vi "Load MICS Tables.vi"() -> ()   [LabVIEW 2010]
doc: "This function is an offline tool for importing MICS Command and Response Tables from Excel. \n\nInstructions\n1) Copy clipboard from Excel to Import Control.\n2) Run VI.\n3) Edit - Make Current Values Defaults.\n4) Save VI.\n5) Copy tables to new VIs."
panel:
  out "error out":errorcluster
  in  "error in":errorcluster
  in  "Table 2":string[][](table)=[["255", "0xFF", "COMMAND ACCEPTED", "The received command (identified in the response) was processed and performed without error. Any data to be returned as a result of the command completion is present in the response."], ["0", "0x00", "INVALID EXID", "The External ID contained in the command is for an external device the xPG has not been configured to process commands from."], ["1", "0x01", "INVALID COMMAND", "The Token in the received command is invalid/unknown to the xPG."], ["2", "0x02", "INVALID PARAM", "A parameter provided with the received command has been determined to be invalid and prohibits further processing of the command."], ["3", "0x03", "BUSY", "The xPG cannot execute the received command while in its present operational state.  Examples include: * Selecting program while stim on * Restoring program defaults while stim on * Writing to flash while stim on [CP commands] "], ["16", "0x10", "COMMAND NOT VALID WHILE IDLE", "The command is not valid when stimulation is not active.  (This code generally applies to commands that are used to modify stimulation.)"], ["17", "0x11", "COMMAND NOT VALID WHILE RAMPING", "The command is not valid when the xPG is ramping the stimulus amplitude immediately after turning stimulation on.  (This code generally applies to commands that are used to modify stimulation parameters)"], ["18", "0x12", "COMMAND LOCKED OUT (temporary)", "The command is temporarily locked out. (This code generally applies to commands that are used to modify stimulation, resulting in an increase in stimulation energy)"], ["19", "0x13", "DEPRECATED", ""], ["32", "0x20", "PROGRAM NOT VALID", "The command cannot be executed because the program definition is not valid.  A way to delete a program is to set it not valid.  Then when IPG returns valid programs bitmap it will not be listed as available."], ["33", "0x21", "PROGRAM DISABLED", "The command cannot be executed because the program definition has been disabled, due to a hardware issue."], ["34", "0x22", "BATTERY TOO LOW", "The xPG Stimulation command to turn stimulation on cannot be executed because the battery level is too low for safe stimulation.  IPG could have said battery was OK, but then dropped below threshold since having last sent status.  "], ["35", "0x23", "DEPRECATED –  Use 0x03 BUSY. ", ""], ["36", "0x24", "NO PROGRAM SELECTED", "The requested command (only in response to stim on) cannot be executed because no program is presently selected."], ["37", "0x25", "BOOST CONVERTER STARTUP FAILED", "Stimulation cannot be started because the high voltage boost converter did not initialize correctly."], ["38", "0x26", "PULSE GUARD CHECK FAILED", "Stimulation cannot be started because the pulse guard circuit check failed."], ["39", "0x27", "STIMULATION POWER ON FAILED", "Stimulation cannot be started because the stimulation chip failed to power up correctly."], ["40", "0x28", "ACTIVE RECOVERY DISABLED", "Stimulation cannot be started because automatic waveform adjustment failed."], ["41", "0x29", "DEPRECATED – Use 0x36 MOD VIOLATES ELECTRODE CHARGE DENSITY LIMIT", ""], ["42", "0x2A", "DEPRECATED – Use 0x02 INVALID PARAM.", ""], ["43", "0x2B", "DEPRECATED – USE 0x02 INVALID PARAM.", ""], ["44", "0x2C", "DEPRECATED – Use 0x02 INVALID PARAM.", ""], ["45", "0x2D", "DEPRECATED – Use 0x02 INVALID PARAM.", ""], ["46", "0x2E", "SETUP ERROR, BAD STIM ASIC READ-BACK", "While attempting to set-up the stim ASIC for output, the verification data read-back of certain registers did not match the set-up data. "], ["47", "0x2F", "SETUP ERROR, BAD POWER ASIC READ-BACK", "While attempting to configure the power ASIC, the verification data read-back of certain registers did not match the set-up data."], ["48", "0x30", "DEPRECATED – Not Used.", ""], ["49", "0x31", "ALL AMPLITUDES AT MINIMUM", "The Decrement Program Amplitude command cannot be executed because all pulse amplitudes are the minimum allowed setting."], ["50", "0x32", "ALL AMPLITUDES AT MAXIMUM", "The Increment Program Amplitude command cannot be executed because all pulse amplitudes are the maximum allowed setting."], ["51", "0x33", "PULSE NOT VALID", "The command to modify the specified pulse amplitude or pulse width cannot be executed because the pulse in not defined in the program that is running."], ["52", "0x34", "PULSE WIDTH EXCEEDS LIMITS", "The requested pulse width modification command cannot be executed because it would exceed the programmed pulse width limits for the specified pulse."], ["53", "0x35", "DEPRECATED - Use 0x02 INVALID PARAM.", ""], ["54", "0x36", "MOD VIOLATES ELECTRODE CHARGE DENSITY LIMIT", "The requested pulse output modification cannot be executed because it would violate the charge density limit for one or more of the selected electrode channels."], ["55", "0x37", "MOD VIOLATES ELECTRODE CURRENT DENSITY LIMIT", "The requested pulse output modification cannot be executed because it would violate the current density limit for one or more of the selected electrode channels."], ["56", "0x38", "PULSE WIDTH FREQUENCY CONFLICT", "* The requested pulse width increase cannot be executed because the program cannot be implemented at the specified program frequency. * The requested program frequency increase cannot be executed because the program cannot be implemented with the specified pulse widths. * The requested Test Pulse will not fit in the selected program period. * The requested pulse output requires active recovery, but the KrecsEnabledBitMap in the Pulse Constants is 0 (no krecs enabled). * The requested pulse output requires active recovery, but there are no krecs enabled (KrecsEnabledBitMap in Pulse Constants) that will fit the selected program period. "], ["57", "0x39", "DEPRECATED – Use PULSE WIDTH FREQUENCY CONFLICT", ""], ["58", "0x3A", "FREQUENCY MOD NOT ALLOWED", "The requested program frequency change is not allowed per the program definition.  (This could be because the specified frequency is not allowed or there is no frequency index lower or higher than the present index allowed.)"], ["59", "0x3B", "PULSE AMPLITUDE EXCEEDS LIMITS", "The requested pulse amplitude change cannot be executed because it would exceed the allowed limits for the specified pulse."], ["60", "0x3C", "DEPRECATED – Command n long exists", ""], ["64", "0x40", "TIMED OUT", "The operation requested timed out waiting for hardware to respond.  This response includes when an ADC read fails or when background impedance check fails to respond with a value."], ["85", "0x55", "CHARGING CONTROL ERROR", "An error occurred reading the temperature or battery level."], ["96", "0x60", "DATA CORRUPTED", "The requested Get Data command failed, or the requested data was detected as corrupt."], ["97", "0x61", "PROGRAM DEFINITION CORRUPTED", "The data integrity check for the program definition data for the requested program failed. IPG should set active error to PROGRAM DEFINITION CORRUPTED"], ["98", "0x62", "PROGRAM ACTIVE SETTINGS CORRUPTED", "The data integrity check for the active settings for the requested program failed.  IPG should set active error to PROGRAM ACTIVE SETTINGS CORRUPTED.  IPG will also return that active settings to default settings."], ["99", "0x63", "PROGRAM CONSTANTS CORRUPTED", "The data integrity check for the Program Constants data failed.  xPG should set active error to CRITICAL NV DATA CORRUPTED."], ["100", "0x64", "PULSE CONSTANTS CORRUPTED", "The data integrity check for the Pulse Constants data failed.  xPG should set active error to CRITICAL NV DATA CORRUPTED."], ["101", "0x65", "CHANNEL CALIBRATIONS CORRUPTED", "The data integrity check for the Channel Calibrations data failed.  xPG should set active error to CRITICAL NV DATA CORRUPTED."], ["102", "0x66", "LEAD LIMITS CORRUPTED", "The data integrity check for the Lead Limits data failed.  xPG should set active error to CRITICAL NV DATA CORRUPTED."], ["103", "0x67", "STIM ASIC HV CALIBRATIONS CORRUPTED", "The data integrity check for the Stim Asic HV Calibrations data failed.  xPG should set active error to CRITICAL NV DATA CORRUPTED."], ["104", "0x68", "RAMP TIME CORRUPTED", "The data integrity check for the Ramp Time failed.  xPG should set active error to CRITICAL NV DATA CORRUPTED."], ["105", "0x69", "DEPRECATED", ""], ["106", "0x6A", "DEPRECATED – Not Used", ""], ["112", "0x70", "FEATURE NOT ENABLED", "The requested feature is not presently enabled."], ["113", "0x71", "DEPRECATED - Use 0x02 INVALID PARAM.", ""], ["114", "0x72", "DEPRECATED - Use 0x02 INVALID PARAM.", ""], ["115", "0x73", "DEPRECATED – Use 0x03 BUSY.", ""], ["116", "0x74", "DEPRECATED – Use 0x38 PULSE WIDTH FREQUENCY CONFLICT", ""], ["117", "0x75", "DEPRECATED – Use 0x38 PULSE WIDTH FREQUENCY CONFLICT", ""], ["118", "0x76", "DEPRECATED – Use 0x38 PULSE WIDTH FREQUENCY CONFLICT", ""], ["119", "0x77", "WRITE FAILED", "The command failed while attempting to write data to memory or registers. Writes to flash shall use more specific error codes from the range below."], ["120", "0x78", "READ FAILED", "The command failed while attempting to read data to memory or registers. Reads to flash shall use more specific error codes from the range below."], ["121", "0x79", "DEPRECATED – Not Used", ""], ["128", "0x80", "DEPRECATED – Not Used", ""], ["129", "0x81", "BACKGROUND IMPEDANCE CHECK FAILED", "Pre-stimulation background impedance checks have failed.  This shall result in a Category 2 Error being reported."], ["130", "0x82", "BASIC OUTPUT CHECK FAILED", "Pre-stimulation basic output checks have failed.  This shall result in a Category 2 Error being reported."], ["131", "0x83", "STIM FAILED UNKNOWN SOFTWARE ERROR", "Stimulation has failed because of a software logic error.  Stimulation cannot be started."], ["132", "0x84", "STIMULATION FAILED – SEVERE ERROR EXISTS", "Stimulation has failed because a Category 1 error exists.  Stimulation cannot be started if such an error exists."], ["133", "0x85", "DEPRECATED – Not Used", ""], ["176", "0xB0", "FLASH ERROR INVALID ADDRESS", "Illegal flash address segment write.  The requested programming command failed while attempting to save data to the xPG’s non-volatile memory."], ["177", "0xB1", "FLASH ERROR SEGMENT BOUNDARY", "Requested flash address write overlaps segment boundary.  The requested programming command failed while attempting to save data to the xPG’s non-volatile memory."], ["178", "0xB2", "DEPRECATED – Use 0xB0 FLASH ERROR INVALID ADDRESS", "Invalid flash address reported while preparing for erasing segment.  The requested programming command failed while attempting to save data to the xPG’s non-volatile memory."], ["179", "0xB3", "FLASH ERASE ERROR FLASH CONTROLLER BUSY", "Flash controller unexpectedly reported busy while preparing for segment erase.  The requested programming command failed while attempting to save data to the xPG’s non-volatile memory."], ["180", "0xB4", "FLASH ERASE ERROR FLASH CONTROLLER SETUP", "Firmware setup error reported while preparing for segment erase.  The requested programming command failed while attempting to save data to the xPG’s non-volatile memory."], ["181", "0xB5", "FLASH ERASE ERROR TIMEOUT", "Busy bit timeout reported while waiting for segment erase. The requested programming command failed while attempting to save data to the xPG’s non-volatile memory."], ["182", "0xB6", "FLASH ERASE ERROR FAIL FLAG", "Fail flag set during segment erase.  The requested programming command failed while attempting to save data to the xPG’s non-volatile memory."], ["183", "0xB7", "FLASH ERASE ERROR ACCESS VIOLATION FLAG", "Access violation reported while attempting to erase flash.  The requested programming command failed while attempting to save data to the xPG’s non-volatile memory."], ["184", "0xB8", "FLASH ERASE ERROR BAD ERASE", "Segment not erased and segment erase reported as completed.  The requested programming command failed while attempting to save data to the xPG’s non-volatile memory."], ["192", "0xC0", "DEPRECATED – Use 0xB0 FLASH ERROR INVALID ADDRESS", ""], ["193", "0xC1", "FLASH WRITE ERROR FLASH CONTROLLER BUSY", "The flash controller reports unexpectedly busy while preparing for block write.  The requested programming command failed while attempting to save data to the xPG’s non-volatile memory."], ["194", "0xC2", "FLASH WRITE ERROR FLASH CONTROLLER SETUP", "A firmware setup error occurred while preparing for block write.  The requested programming command failed while attempting to save data to the xPG’s non-volatile memory."], ["195", "0xC3", "FLASH WORD WRITE ERROR TIMEOUT", "Wait bit timeout occurred while writing word to flash memory.  The requested programming command failed while attempting to save data to the xPG’s non-volatile memory."], ["196", "0xC4", "FLASH  WORD WRITE ERROR FAIL FLAG", "Flash fail flag set while writing word to flash memory.  The requested programming command failed while attempting to save data to the xPG’s non-volatile memory."], ["197", "0xC5", "FLASH WORD WRITE ERROR ACCESS VIOLATION", "Access violation reported while writing word to flash memory.  The requested programming command failed while attempting to save data to the xPG’s non-volatile memory."], ["198", "0xC6", "FLASH BLOCK WRITE ERROR TIMEOUT", "Wait bit timeout occurred while writing block to flash memory.  The requested programming command failed while attempting to save data to the xPG’s non-volatile memory."], ["199", "0xC7", "FLASH  BLOCK WRITE ERROR FAIL FLAG", "Flash fail flag set while writing block to flash memory.  The requested programming command failed while attempting to save data to the xPG’s non-volatile memory."], ["200", "0xC8", "FLASH BLOCK WRITE ERROR ACCESS VIOLATION", "Access violation reported while writing block to flash memory.  The requested programming command failed while attempting to save data to the xPG’s non-volatile memory."], ["201", "0xC9", "FLASH WRITE ERROR BAD WRITE", "After segment write completed, the flash destination data did not match the source data.  The requested programming command failed while attempting to save data to the xPG’s non-volatile memory."], ["202", "0xCA", "RESERVED – Not Used.", ""], ["203", "0xCB", "RESERVED – Not Used.", ""], ["204", "0xCC", "RESERVED – Not Used.", ""], ["205", "0xCD", "RESERVED – Not Used.", ""], ["206", "0xCE", "RESERVED – Not Used.", ""], ["207", "0xCF", "RESERVED – Not Used.", ""], ["-1", "Default", "ANY ERROR NOT LISTED HEREIN", "Undefined and unexpected.   "]]
  in  "Excel Clipboard to Import 2":string="255\t0xFF\tCOMMAND ACCEPTED\tThe received command (identified in the response) was processed and performed without error. Any data to be returned as a result of the command completion is present in the response.\n0\t0x00\tINVALID EXID\tThe External ID contained in the command is for an external device the xPG has not been configured to process commands from.\n1\t0x01\tINVALID COMMAND\tThe Token in the received command is invalid/unknown to the xPG.\n2\t0x02\tINVALID PARAM\tA parameter provided with the received command has been determined to be invalid and prohibits further processing of the command.\n3\t0x03\tBUSY\tThe xPG cannot execute the received command while in its present operational state.  Examples include: * Selecting program while stim on * Restoring program defaults while stim on * Writing to flash while stim on [CP commands] \n16\t0x10\tCOMMAND NOT VALID WHILE IDLE\tThe command is not valid when stimulation is not active.  (This code generally applies to commands that are used to modify stimulation.)\n17\t0x11\tCOMMAND NOT VALID WHILE RAMPING\tThe command is not valid when the xPG is ramping the stimulus amplitude immediately after turning stimulation on.  (This code generally applies to commands that are used to modify stimulation parameters)\n18\t0x12\tCOMMAND LOCKED OUT (temporary)\tThe command is temporarily locked out. (This code generally applies to commands that are used to modify stimulation, resulting in an increase in stimulation energy)\n19\t0x13\tDEPRECATED\t\n32\t0x20\tPROGRAM NOT VALID\tThe command cannot be executed because the program definition is not valid.  A way to delete a program is to set it not valid.  Then when IPG returns valid programs bitmap it will not be listed as available.\n33\t0x21\tPROGRAM DISABLED\tThe command cannot be executed because the program definition has been disabled, due to a hardware issue.\n34\t0x22\tBATTERY TOO LOW\tThe xPG Stimulation command to turn stimulation on cannot be executed because the battery level is too low for safe stimulation.  IPG could have said battery was OK, but then dropped below threshold since having last sent status.  \n35\t0x23\tDEPRECATED –  Use 0x03 BUSY. \t\n36\t0x24\tNO PROGRAM SELECTED\tThe requested command (only in response to stim on) cannot be executed because no program is presently selected.\n37\t0x25\tBOOST CONVERTER STARTUP FAILED\tStimulation cannot be started because the high voltage boost converter did not initialize correctly.\n38\t0x26\tPULSE GUARD CHECK FAILED\tStimulation cannot be started because the pulse guard circuit check failed.\n39\t0x27\tSTIMULATION POWER ON FAILED\tStimulation cannot be started because the stimulation chip failed to power up correctly.\n40\t0x28\tACTIVE RECOVERY DISABLED\tStimulation cannot be started because automatic waveform adjustment failed.\n41\t0x29\tDEPRECATED – Use 0x36 MOD VIOLATES ELECTRODE CHARGE DENSITY LIMIT\t\n42\t0x2A\tDEPRECATED – Use 0x02 INVALID PARAM.\t\n43\t0x2B\tDEPRECATED – USE 0x02 INVALID PARAM.\t\n44\t0x2C\tDEPRECATED – Use 0x02 INVALID PARAM.\t\n45\t0x2D\tDEPRECATED – Use 0x02 INVALID PARAM.\t\n46\t0x2E\tSETUP ERROR, BAD STIM ASIC READ-BACK\tWhile attempting to set-up the stim ASIC for output, the verification data read-back of certain registers did not match the set-up data. \n47\t0x2F\tSETUP ERROR, BAD POWER ASIC READ-BACK\tWhile attempting to configure the power ASIC, the verification data read-back of certain registers did not match the set-up data.\n48\t0x30\tDEPRECATED – Not Used.\t\n49\t0x31\tALL AMPLITUDES AT MINIMUM\tThe Decrement Program Amplitude command cannot be executed because all pulse amplitudes are the minimum allowed setting.\n50\t0x32\tALL AMPLITUDES AT MAXIMUM\tThe Increment Program Amplitude command cannot be executed because all pulse amplitudes are the maximum allowed setting.\n51\t0x33\tPULSE NOT VALID\tThe command to modify the specified pulse amplitude or pulse width cannot be executed because the pulse in not defined in the program that is running.\n52\t0x34\tPULSE WIDTH EXCEEDS LIMITS\tThe requested pulse width modification command cannot be executed because it would exceed the programmed pulse width limits for the specified pulse.\n53\t0x35\tDEPRECATED - Use 0x02 INVALID PARAM.\t\n54\t0x36\tMOD VIOLATES ELECTRODE CHARGE DENSITY LIMIT\tThe requested pulse output modification cannot be executed because it would violate the charge density limit for one or more of the selected electrode channels.\n55\t0x37\tMOD VIOLATES ELECTRODE CURRENT DENSITY LIMIT\tThe requested pulse output modification cannot be executed because it would violate the current density limit for one or more of the selected electrode channels.\n56\t0x38\tPULSE WIDTH FREQUENCY CONFLICT\t* The requested pulse width increase cannot be executed because the program cannot be implemented at the specified program frequency. * The requested program frequency increase cannot be executed because the program cannot be implemented with the specified pulse widths. * The requested Test Pulse will not fit in the selected program period. * The requested pulse output requires active recovery, but the KrecsEnabledBitMap in the Pulse Constants is 0 (no krecs enabled). * The requested pulse output requires active recovery, but there are no krecs enabled (KrecsEnabledBitMap in Pulse Constants) that will fit the selected program period. \n57\t0x39\tDEPRECATED – Use PULSE WIDTH FREQUENCY CONFLICT\t\n58\t0x3A\tFREQUENCY MOD NOT ALLOWED\tThe requested program frequency change is not allowed per the program definition.  (This could be because the specified frequency is not allowed or there is no frequency index lower or higher than the present index allowed.)\n59\t0x3B\tPULSE AMPLITUDE EXCEEDS LIMITS\tThe requested pulse amplitude change cannot be executed because it would exceed the allowed limits for the specified pulse.\n60\t0x3C\tDEPRECATED – Command n long exists\t\n64\t0x40\tTIMED OUT\tThe operation requested timed out waiting for hardware to respond.  This response includes when an ADC read fails or when background impedance check fails to respond with a value.\n85\t0x55\tCHARGING CONTROL ERROR\tAn error occurred reading the temperature or battery level.\n96\t0x60\tDATA CORRUPTED\tThe requested Get Data command failed, or the requested data was detected as corrupt.\n97\t0x61\tPROGRAM DEFINITION CORRUPTED\tThe data integrity check for the program definition data for the requested program failed. IPG should set active error to PROGRAM DEFINITION CORRUPTED\n98\t0x62\tPROGRAM ACTIVE SETTINGS CORRUPTED\tThe data integrity check for the active settings for the requested program failed.  IPG should set active error to PROGRAM ACTIVE SETTINGS CORRUPTED.  IPG will also return that active settings to default settings.\n99\t0x63\tPROGRAM CONSTANTS CORRUPTED\tThe data integrity check for the Program Constants data failed.  xPG should set active error to CRITICAL NV DATA CORRUPTED.\n100\t0x64\tPULSE CONSTANTS CORRUPTED\tThe data integrity check for the Pulse Constants data failed.  xPG should set active error to CRITICAL NV DATA CORRUPTED.\n101\t0x65\tCHANNEL CALIBRATIONS CORRUPTED\tThe data integrity check for the Channel Calibrations data failed.  xPG should set active error to CRITICAL NV DATA CORRUPTED.\n102\t0x66\tLEAD LIMITS CORRUPTED\tThe data integrity check for the Lead Limits data failed.  xPG should set active error to CRITICAL NV DATA CORRUPTED.\n103\t0x67\tSTIM ASIC HV CALIBRATIONS CORRUPTED\tThe data integrity check for the Stim Asic HV Calibrations data failed.  xPG should set active error to CRITICAL NV DATA CORRUPTED.\n104\t0x68\tRAMP TIME CORRUPTED\tThe data integrity check for the Ramp Time failed.  xPG should set active error to CRITICAL NV DATA CORRUPTED.\n105\t0x69\tDEPRECATED\t\n106\t0x6A\tDEPRECATED – Not Used\t\n112\t0x70\tFEATURE NOT ENABLED\tThe requested feature is not presently enabled.\n113\t0x71\tDEPRECATED - Use 0x02 INVALID PARAM.\t\n114\t0x72\tDEPRECATED - Use 0x02 INVALID PARAM.\t\n115\t0x73\tDEPRECATED – Use 0x03 BUSY.\t\n116\t0x74\tDEPRECATED – Use 0x38 PULSE WIDTH FREQUENCY CONFLICT\t\n117\t0x75\tDEPRECATED – Use 0x38 PULSE WIDTH FREQUENCY CONFLICT\t\n118\t0x76\tDEPRECATED – Use 0x38 PULSE WIDTH FREQUENCY CONFLICT\t\n119\t0x77\tWRITE FAILED\tThe command failed while attempting to write data to memory or registers. Writes to flash shall use more specific error codes from the range below.\n120\t0x78\tREAD FAILED\tThe command failed while attempting to read data to memory or registers. Reads to flash shall use more specific error codes from the range below.\n121\t0x79\tDEPRECATED – Not Used\t\n128\t0x80\tDEPRECATED – Not Used\t\n129\t0x81\tBACKGROUND IMPEDANCE CHECK FAILED\tPre-stimulation background impedance checks have failed.  This shall result in a Category 2 Error being reported.\n130\t0x82\tBASIC OUTPUT CHECK FAILED\tPre-stimulation basic output checks have failed.  This shall result in a Category 2 Error being reported.\n131\t0x83\tSTIM FAILED UNKNOWN SOFTWARE ERROR\tStimulation has failed because of a software logic error.  Stimulation cannot be started.\n132\t0x84\tSTIMULATION FAILED – SEVERE ERROR EXISTS\tStimulation has failed because a Category 1 error exists.  Stimulation cannot be started if such an error exists.\n133\t0x85\tDEPRECATED – Not Used\t\n176\t0xB0\tFLASH ERROR INVALID ADDRESS\tIllegal flash address segment write.  The requested programming command failed while attempting to save data to the xPG’s non-volatile memory.\n177\t0xB1\tFLASH ERROR SEGMENT BOUNDARY\tRequested flash address write overlaps segment boundary.  The requested programming command failed while attempting to save data to the xPG’s non-volatile memory.\n178\t0xB2\tDEPRECATED – Use 0xB0 FLASH ERROR INVALID ADDRESS\tInvalid flash address reported while preparing for erasing segment.  The requested programming command failed while attempting to save data to the xPG’s non-volatile memory.\n179\t0xB3\tFLASH ERASE ERROR FLASH CONTROLLER BUSY\tFlash controller unexpectedly reported busy while preparing for segment erase.  The requested programming command failed while attempting to save data to the xPG’s non-volatile memory.\n180\t0xB4\tFLASH ERASE ERROR FLASH CONTROLLER SETUP\tFirmware setup error reported while preparing for segment erase.  The requested programming command failed while attempting to save data to the xPG’s non-volatile memory.\n181\t0xB5\tFLASH ERASE ERROR TIMEOUT\tBusy bit timeout reported while waiting for segment erase. The requested programming command failed while attempting to save data to the xPG’s non-volatile memory.\n182\t0xB6\tFLASH ERASE ERROR FAIL FLAG\tFail flag set during segment erase.  The requested programming command failed while attempting to save data to the xPG’s non-volatile memory.\n183\t0xB7\tFLASH ERASE ERROR ACCESS VIOLATION FLAG\tAccess violation reported while attempting to erase flash.  The requested programming command failed while attempting to save data to the xPG’s non-volatile memory.\n184\t0xB8\tFLASH ERASE ERROR BAD ERASE\tSegment not erased and segment erase reported as completed.  The requested programming command failed while attempting to save data to the xPG’s non-volatile memory.\n192\t0xC0\tDEPRECATED – Use 0xB0 FLASH ERROR INVALID ADDRESS\t\n193\t0xC1\tFLASH WRITE ERROR FLASH CONTROLLER BUSY\tThe flash controller reports unexpectedly busy while preparing for block write.  The requested programming command failed while attempting to save data to the xPG’s non-volatile memory.\n194\t0xC2\tFLASH WRITE ERROR FLASH CONTROLLER SETUP\tA firmware setup error occurred while preparing for block write.  The requested programming command failed while attempting to save data to the xPG’s non-volatile memory.\n195\t0xC3\tFLASH WORD WRITE ERROR TIMEOUT\tWait bit timeout occurred while writing word to flash memory.  The requested programming command failed while attempting to save data to the xPG’s non-volatile memory.\n196\t0xC4\tFLASH  WORD WRITE ERROR FAIL FLAG\tFlash fail flag set while writing word to flash memory.  The requested programming command failed while attempting to save data to the xPG’s non-volatile memory.\n197\t0xC5\tFLASH WORD WRITE ERROR ACCESS VIOLATION\tAccess violation reported while writing word to flash memory.  The requested programming command failed while attempting to save data to the xPG’s non-volatile memory.\n198\t0xC6\tFLASH BLOCK WRITE ERROR TIMEOUT\tWait bit timeout occurred while writing block to flash memory.  The requested programming command failed while attempting to save data to the xPG’s non-volatile memory.\n199\t0xC7\tFLASH  BLOCK WRITE ERROR FAIL FLAG\tFlash fail flag set while writing block to flash memory.  The requested programming command failed while attempting to save data to the xPG’s non-volatile memory.\n200\t0xC8\tFLASH BLOCK WRITE ERROR ACCESS VIOLATION\tAccess violation reported while writing block to flash memory.  The requested programming command failed while attempting to save data to the xPG’s non-volatile memory.\n201\t0xC9\tFLASH WRITE ERROR BAD WRITE\tAfter segment write completed, the flash destination data did not match the source data.  The requested programming command failed while attempting to save data to the xPG’s non-volatile memory.\n202\t0xCA\tRESERVED – Not Used.\t\n203\t0xCB\tRESERVED – Not Used.\t\n204\t0xCC\tRESERVED – Not Used.\t\n205\t0xCD\tRESERVED – Not Used.\t\n206\t0xCE\tRESERVED – Not Used.\t\n207\t0xCF\tRESERVED – Not Used.\t\n-1\tDefault\tANY ERROR NOT LISTED HEREIN\tUndefined and unexpected.   \n"
  in  "Excel Clipboard1 to Import 1":string="1\t0x0001\tGet xPG Status\tTKN_GET_XPG_STATUS\n2\t0x0002\txPG Stimulation\tTKN_XPG_STIMULATION\n3\t0x0003\tSelect Program\tTKN_SELECT_PROGRAM\n4\t0x0004\tIncrement Program Amplitude\tTKN_INC_PRGM_AMPL\n5\t0x0005\tDecrement Program Amplitude\tTKN_DEC_PRGM_AMPL\n6\t0x0006\tGet PoP Constants\tTKN_GET_POP_CONST\n7\t0x0007\tGet PPC Constants\tTKN_GET_PPC CONST\n8\t0x0008\tGet Program Names\tTKN_GET_PRGM_NAMES\n9\t0x0009\tSet Pulse Amplitude\tTKN_SET_PULSE_AMPL\n10\t0x000A\tIncrement Pulse Amplitude\tTKN_INC_PULSE_AMPL\n11\t0x000B\tDecrement Pulse Amplitude\tTKN_DEC_PULSE_AMPL\n12\t0x000C\tGet Pulse Widths\tTKN_GET_PULSE_WIDTHS\n13\t0x000D\tSet Pulse Widths\tTKN_SET_PULSE_WIDTH\n14\t0x000E\tIncrement Pulse Width\tTKN_INC_PULSE_WIDTH\n15\t0x000F\tDecrement Pulse Width\tTKN_DEC_PULSE_WIDTH\n16\t0x0010\tGet Program Frequency\tTKN_GET_PRGM_FREQ\n17\t0x0011\tSet Program Frequency\tTKN_SET_PRGM_FREQ\n18\t0x0012\tIncrement Program Frequency\tTKN_INC_PRGM_FREQ\n19\t0x0013\tDecrement Program Frequency\tTKN_DEC_PRGM_FREQ\n20\t0x0014\tInject Event\tTKN_INJECT_EVENT\n21\t0x0015\tCharging Control\tTKN_CHARGING_CONTROL\n22\t0x0016\tGet xPG Identity\tTKN_GET_XPG_IDENTITY\n23\t0x0017\tSet xPG Identity\tTKN_SET_XPG_IDENTITY\n24\t0x0018\tRestore Program Defaults\tTKN_RESTORE_DEFAULTS\n25\t0x0019\tGet Program Definition\tTKN_GET_PRGM_DEF\n26\t0x001A\tSet Program Definition\tTKN_SET_PRGM_DEF\n27\t0x001B\tGet Program Constants\tTKN_GET_PRGM_CONST\n28\t0x001C\tSet Program Constants\tTKN_SET_PRGM_CONST\n29\t0x001D\tGet Configurable Device Parameters\tTKN_GET_CONFIG_PARAMS\n30\t0x001E\tSet Configurable Device Parameters\tTKN_SET_CONFIG_PARAMS\n31\t0x001F\tGet Pulse Constants\tTKN_GET_PULSE_CONSTANTS\n32\t0x0020\tSet Pulse Constants\tTKN_SET_PULSE_CONSTANTS\n33\t0x0021\tGet Lead Limits\tTKN_GET_LEAD_LIMITS\n34\t0x0022\tSet Lead Limits\tTKN_SET_LEAD_LIMITS\n35\t0x0023\tGet Channel Calibrations\tTKN_GET_CHANNEL_CALS\n36\t0x0024\tSet Channel Calibrations\tTKN_SET_CHANNEL_CALS\n37\t0x0025\t(reserved)\tRESERVED_37\n38\t0x0026\t(reserved)\tRESERVED_38\n39\t0x0027\t(reserved)\tRESERVED_39\n40\t0x0028\t(reserved)\tRESERVED_40\n41\t0x0029\t(reserved)\tRESERVED_41\n42\t0x002A\t(reserved)\tRESERVED_42\n43\t0x002B\tGet Stim Asic HV Calibrations\tTKN_GET_HV_CALS\n44\t0x002C\tSet Stim Asic HV Calibrations\tTKN_SET_HV_CALS\n45\t0x002D\t(reserved)\tRESERVED_45\n46\t0x002E\t(reserved)\tRESERVED_46\n47\t0x002F\tGet CP Data\tTKN_GET_CP_DATA\n48\t0x0030\tSet CP Data\tTKN_SET_CP_DATA\n49\t0x0031\tClear Log\tTKN_CLEAR_LOG\n50\t0x0032\tRead Log\tTKN_READ_LOG\n51\t0x0033\tAppend Log\tTKN_APPEND_LOG\n52\t0x0034\t(reserved)\tRESERVED_52\n53\t0x0035\t(reserved)\tRESERVED_53\n54\t0x0036\tImpedance Measurement\tTKN_IMP_MEAS\n55\t0x0037\tEnter Storage Mode\tTKN_STORAGE\n56\t0x0038\tEcho Short\tTKN_ECHO_SHORT\n57\t0x0039\tEcho Long\tTKN_ECHO_LONG\n58\t0x003A\tGet General Calibration\tTKN_GET_GEN_CAL\n59\t0x003B\tSet General Calibration\tTKN_SET_GEN_CAL\n60\t0x003C\tGet Trim List\tTKN_GET_TRIM_LIST\n61\t0x003D\tSet Trim List\tTKN_SET_TRIM_LIST\n62\t0x003E\tGet Counter\tTKN_GET_COUNTER\n63\t0x003F\tSet Counter\tTKN_SET_COUNTER\n64\t0x0040\tGet Test Stimulation\tTKN_GET_TEST_STIM\n65\t0x0041\tSet Test Stimulation\tTKN_SET_TEST_STIM\n66\t0x0042\tGet Titration Stimulation\tTKN_GET_TITR_STIM\n67\t0x0043\tSet Titration Stimulation\tTKN_SET_TITR_STIM\n68\t0x0044\tGet Ramp Time\tTKN_GET_RAMP_TIME\n69\t0x0045\tSet Ramp Time\tTKN_SET_RAMP_TIME\n70\t0x0046\tGet VBAT\tTKN_GET_VBAT\n71\t0x0047\tSet Software Description Block\tTKN_SET_SDB\n72\t0x0048\tGet Software Description Block\tTKN_GET_SDB\n73\t0x0049\tWrite Memory\tTKN_WRITE_MEMORY\n74\t0x004A\tRead Memory\tTKN_READ_MEMORY\n75\t0x004B\tReset xPG\tTKN_RESET\n76\t0x004C\tErase Flash Block\tTKN_ERASE_FLASH_BLOCK\n77\t0x004D\tWrite Vectors\tTKN_WRITE_VECTORS\n78\t0x004E\tRead Vectors\tTKN_READ_VECTORS\n79\t0x004F\tDiagnostic Data\tTKN_DIAG_DATA\n80\t0x0050\tSet Background Impedance\tTKN_SET_BG_IMPEDANCE\n81\t0x0051\tGet Background Impedance\tTKN_GET_BG_IMPEDANCE\n82\t0x0052\tSet Test Waveform\tTKN_SET_TEST_WAVEFORM\n83\t0x0053\tCalibrate Channel\tTKN_CALIBRATE_CHANNEL\n84\t0x0054\tGet Log Range\tTKN_GET_LOG_RANGE\n85\t0x0055\t(reserved)\tRESERVED_85\n86\t0x0056\t(reserved)\tRESERVED_86\n87\t0x0057\tMICS Options\tTKN_MICS_OPTIONS\n88\t0x0058\tPair PPC\tTKN_PAIR_PPC\n89\t0x0059\tPair PoP\tTKN_PAIR_POP\n90\t0x005A\tStop Bootloader\tTKN_STOP_BOOTLOADER\n91\t0x005B\tTune MICS\tTKN_MICS_TUNE\n92\t0x005C\tMICS Diagnostics\tTKN_MICS_DIAGNOSTICS\n32682\t0x7FAA\tUndefined\tTKN_UNDEFINED\n"
  in  "Table 1":string[][](table)=[["1", "0x0001", "Get xPG Status", "TKN_GET_XPG_STATUS"], ["2", "0x0002", "xPG Stimulation", "TKN_XPG_STIMULATION"], ["3", "0x0003", "Select Program", "TKN_SELECT_PROGRAM"], ["4", "0x0004", "Increment Program Amplitude", "TKN_INC_PRGM_AMPL"], ["5", "0x0005", "Decrement Program Amplitude", "TKN_DEC_PRGM_AMPL"], ["6", "0x0006", "Get PoP Constants", "TKN_GET_POP_CONST"], ["7", "0x0007", "Get PPC Constants", "TKN_GET_PPC CONST"], ["8", "0x0008", "Get Program Names", "TKN_GET_PRGM_NAMES"], ["9", "0x0009", "Set Pulse Amplitude", "TKN_SET_PULSE_AMPL"], ["10", "0x000A", "Increment Pulse Amplitude", "TKN_INC_PULSE_AMPL"], ["11", "0x000B", "Decrement Pulse Amplitude", "TKN_DEC_PULSE_AMPL"], ["12", "0x000C", "Get Pulse Widths", "TKN_GET_PULSE_WIDTHS"], ["13", "0x000D", "Set Pulse Widths", "TKN_SET_PULSE_WIDTH"], ["14", "0x000E", "Increment Pulse Width", "TKN_INC_PULSE_WIDTH"], ["15", "0x000F", "Decrement Pulse Width", "TKN_DEC_PULSE_WIDTH"], ["16", "0x0010", "Get Program Frequency", "TKN_GET_PRGM_FREQ"], ["17", "0x0011", "Set Program Frequency", "TKN_SET_PRGM_FREQ"], ["18", "0x0012", "Increment Program Frequency", "TKN_INC_PRGM_FREQ"], ["19", "0x0013", "Decrement Program Frequency", "TKN_DEC_PRGM_FREQ"], ["20", "0x0014", "Inject Event", "TKN_INJECT_EVENT"], ["21", "0x0015", "Charging Control", "TKN_CHARGING_CONTROL"], ["22", "0x0016", "Get xPG Identity", "TKN_GET_XPG_IDENTITY"], ["23", "0x0017", "Set xPG Identity", "TKN_SET_XPG_IDENTITY"], ["24", "0x0018", "Restore Program Defaults", "TKN_RESTORE_DEFAULTS"], ["25", "0x0019", "Get Program Definition", "TKN_GET_PRGM_DEF"], ["26", "0x001A", "Set Program Definition", "TKN_SET_PRGM_DEF"], ["27", "0x001B", "Get Program Constants", "TKN_GET_PRGM_CONST"], ["28", "0x001C", "Set Program Constants", "TKN_SET_PRGM_CONST"], ["29", "0x001D", "Get Configurable Device Parameters", "TKN_GET_CONFIG_PARAMS"], ["30", "0x001E", "Set Configurable Device Parameters", "TKN_SET_CONFIG_PARAMS"], ["31", "0x001F", "Get Pulse Constants", "TKN_GET_PULSE_CONSTANTS"], ["32", "0x0020", "Set Pulse Constants", "TKN_SET_PULSE_CONSTANTS"], ["33", "0x0021", "Get Lead Limits", "TKN_GET_LEAD_LIMITS"], ["34", "0x0022", "Set Lead Limits", "TKN_SET_LEAD_LIMITS"], ["35", "0x0023", "Get Channel Calibrations", "TKN_GET_CHANNEL_CALS"], ["36", "0x0024", "Set Channel Calibrations", "TKN_SET_CHANNEL_CALS"], ["37", "0x0025", "(reserved)", "RESERVED_37"], ["38", "0x0026", "(reserved)", "RESERVED_38"], ["39", "0x0027", "(reserved)", "RESERVED_39"], ["40", "0x0028", "(reserved)", "RESERVED_40"], ["41", "0x0029", "(reserved)", "RESERVED_41"], ["42", "0x002A", "(reserved)", "RESERVED_42"], ["43", "0x002B", "Get Stim Asic HV Calibrations", "TKN_GET_HV_CALS"], ["44", "0x002C", "Set Stim Asic HV Calibrations", "TKN_SET_HV_CALS"], ["45", "0x002D", "(reserved)", "RESERVED_45"], ["46", "0x002E", "(reserved)", "RESERVED_46"], ["47", "0x002F", "Get CP Data", "TKN_GET_CP_DATA"], ["48", "0x0030", "Set CP Data", "TKN_SET_CP_DATA"], ["49", "0x0031", "Clear Log", "TKN_CLEAR_LOG"], ["50", "0x0032", "Read Log", "TKN_READ_LOG"], ["51", "0x0033", "Append Log", "TKN_APPEND_LOG"], ["52", "0x0034", "(reserved)", "RESERVED_52"], ["53", "0x0035", "(reserved)", "RESERVED_53"], ["54", "0x0036", "Impedance Measurement", "TKN_IMP_MEAS"], ["55", "0x0037", "Enter Storage Mode", "TKN_STORAGE"], ["56", "0x0038", "Echo Short", "TKN_ECHO_SHORT"], ["57", "0x0039", "Echo Long", "TKN_ECHO_LONG"], ["58", "0x003A", "Get General Calibration", "TKN_GET_GEN_CAL"], ["59", "0x003B", "Set General Calibration", "TKN_SET_GEN_CAL"], ["60", "0x003C", "Get Trim List", "TKN_GET_TRIM_LIST"], ["61", "0x003D", "Set Trim List", "TKN_SET_TRIM_LIST"], ["62", "0x003E", "Get Counter", "TKN_GET_COUNTER"], ["63", "0x003F", "Set Counter", "TKN_SET_COUNTER"], ["64", "0x0040", "Get Test Stimulation", "TKN_GET_TEST_STIM"], ["65", "0x0041", "Set Test Stimulation", "TKN_SET_TEST_STIM"], ["66", "0x0042", "Get Titration Stimulation", "TKN_GET_TITR_STIM"], ["67", "0x0043", "Set Titration Stimulation", "TKN_SET_TITR_STIM"], ["68", "0x0044", "Get Ramp Time", "TKN_GET_RAMP_TIME"], ["69", "0x0045", "Set Ramp Time", "TKN_SET_RAMP_TIME"], ["70", "0x0046", "Get VBAT", "TKN_GET_VBAT"], ["71", "0x0047", "Set Software Description Block", "TKN_SET_SDB"], ["72", "0x0048", "Get Software Description Block", "TKN_GET_SDB"], ["73", "0x0049", "Write Memory", "TKN_WRITE_MEMORY"], ["74", "0x004A", "Read Memory", "TKN_READ_MEMORY"], ["75", "0x004B", "Reset xPG", "TKN_RESET"], ["76", "0x004C", "Erase Flash Block", "TKN_ERASE_FLASH_BLOCK"], ["77", "0x004D", "Write Vectors", "TKN_WRITE_VECTORS"], ["78", "0x004E", "Read Vectors", "TKN_READ_VECTORS"], ["79", "0x004F", "Diagnostic Data", "TKN_DIAG_DATA"], ["80", "0x0050", "Set Background Impedance", "TKN_SET_BG_IMPEDANCE"], ["81", "0x0051", "Get Background Impedance", "TKN_GET_BG_IMPEDANCE"], ["82", "0x0052", "Set Test Waveform", "TKN_SET_TEST_WAVEFORM"], ["83", "0x0053", "Calibrate Channel", "TKN_CALIBRATE_CHANNEL"], ["84", "0x0054", "Get Log Range", "TKN_GET_LOG_RANGE"], ["85", "0x0055", "(reserved)", "RESERVED_85"], ["86", "0x0056", "(reserved)", "RESERVED_86"], ["87", "0x0057", "MICS Options", "TKN_MICS_OPTIONS"], ["88", "0x0058", "Pair PPC", "TKN_PAIR_PPC"], ["89", "0x0059", "Pair PoP", "TKN_PAIR_POP"], ["90", "0x005A", "Stop Bootloader", "TKN_STOP_BOOTLOADER"], ["91", "0x005B", "Tune MICS", "TKN_MICS_TUNE"], ["92", "0x005C", "MICS Diagnostics", "TKN_MICS_DIAGNOSTICS"], ["32682", "0x7FAA", "Undefined", "TKN_UNDEFINED"]]
  # "SWEX 0085 Rev 1.11"
  # "SWEX 0091  Rev 1.8"
  # "Instructions\n1) Copy clipboard from Excel to Import Control.\n2) Run VI.\n3) Edit - Make Current Values Defaults.\n4) Save VI.\n5) Copy tables to new VIs."
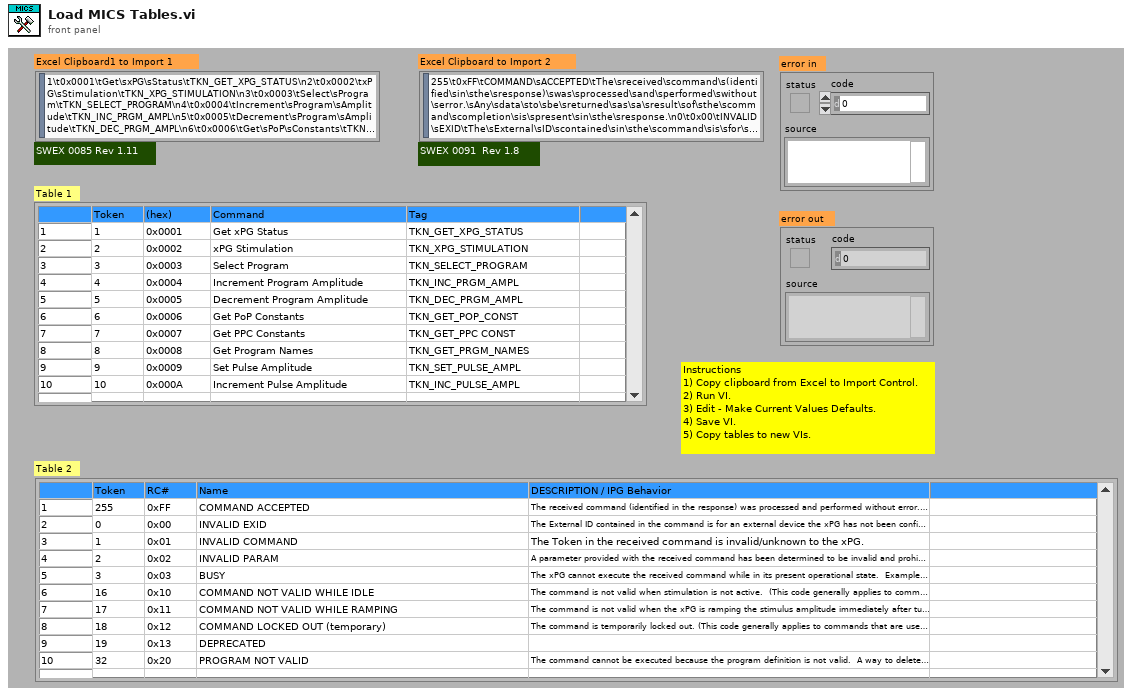
[diagram p1: front panel]
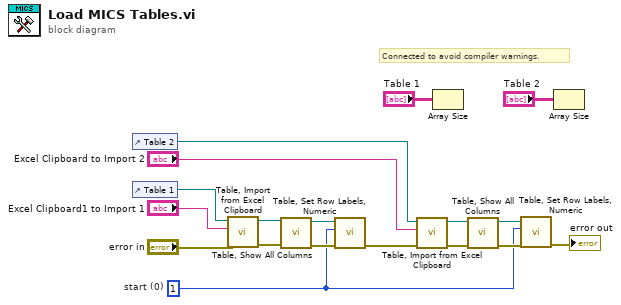
[diagram p0: block diagram]
diagram:
  w3 = 1  # start (0)
  # "Connected to avoid compiler warnings."
  n1 = control-ref of="Table 2"() -> (w5:refnum<vi>)
  n2 = control-ref of="Table 1"() -> (w17:refnum<vi>)
  n3 = call "Table, Import from Excel Clipboard.vi"("error in"="error in", "Excel Clipboard to Import"="Excel Clipboard1 to Import 1", "Tbl Refnum"=w17) -> ("error out"=w15:errorcluster, "Tbl Refnumout"=w16:refnum<vi>)  [unwired: 7 in]
  n4 = call "Table, Show All Columns.vi"("error in"=w15, "Tbl Refnum"=w16) -> ("error out"=w13:errorcluster, "Tbl Refnum out"=w12:refnum<vi>)  [unwired: 8 in]
  n5 = call "Table, Set Row Labels, Numeric.vi"("error in"=w13, "start (0)"=w3, "Tbl Refnum"=w12) -> ("error out"=w11:errorcluster)  [unwired: 7 in, 1 out]
  n6 = call "Table, Import from Excel Clipboard.vi"("error in"=w11, "Excel Clipboard to Import"="Excel Clipboard to Import 2", "Tbl Refnum"=w5) -> ("error out"=w10:errorcluster, "Tbl Refnumout"=w2:refnum<vi>)  [unwired: 7 in]
  n7 = Array Size(array="Table 1") -> ()  [unwired: 1 out]
  n8 = call "Table, Show All Columns.vi"("error in"=w10, "Tbl Refnum"=w2) -> ("error out"=w9:errorcluster, "Tbl Refnum out"=w1:refnum<vi>)  [unwired: 8 in]
  n9 = call "Table, Set Row Labels, Numeric.vi"("error in"=w9, "start (0)"=w3, "Tbl Refnum"=w1) -> ("error out"=→"error out":errorcluster)  [unwired: 7 in, 1 out]
  n10 = Array Size(array="Table 2") -> ()  [unwired: 1 out]
